vi "1.3主程序.vi"() -> ()   [LabVIEW 2016]
panel:
  out "与100相加后开方":dbl
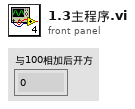
[diagram p1: front panel]
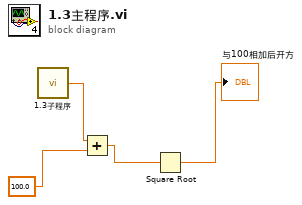
[diagram p0: block diagram]
diagram:
  n1 = call "1.3子程序.vi"() -> ("数值"=w4:dbl)
  n2 = Add(x=w4, y=100.0) -> (x+y=w2:dbl)
  n3 = Square Root(x=w2) -> (sqrt(x)=→"与100相加后开方":dbl)
